vi "NI VeriStand - Get All Waveforms.vi"(8 "error in":errorcluster, 11 "Section Ref in":T1 format="%.0x") -> (0 "error out":errorcluster, 2 "Waveform Refs":T1[](array[typedef]) format="%.0x", 3 "Section Ref out":T1 format="%.0x", 4 "Found":bool)   [LabVIEW 2020, in "Custom Device Utility Library.lvlib"]
doc: "Gets an array of references for all the waveforms within the custom-device section specified by <B>Section Ref in</B>.\n\nThis VI performs a depth-first deep search."
uses:
  <vilib>/NI VeriStand/Custom Device Tools/Custom Device Utility Library/Custom Device Utility Library.lvlib
  <vilib>/NI VeriStand/Custom Device API/Custom Device Item Ref.ctl
  <vilib>/NI VeriStand/Custom Device API/Custom Device API.lvlib
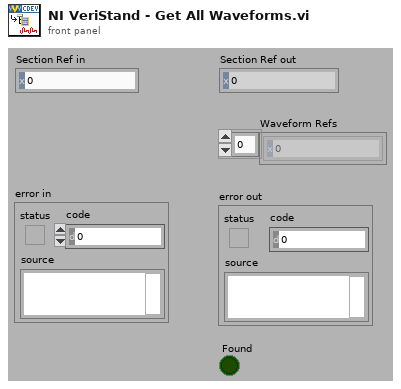
[diagram p1: front panel]
types:
  T1 = typedef "Custom Device API.lvlib/Custom Device Item Ref.ctl" = u64
  T2 = typedef "Custom Device API.lvlib/Custom Device Item Info.ctl" = cluster{"Name":string, "Is Channel":bool, "GUID":string, "Is Waveform":bool}
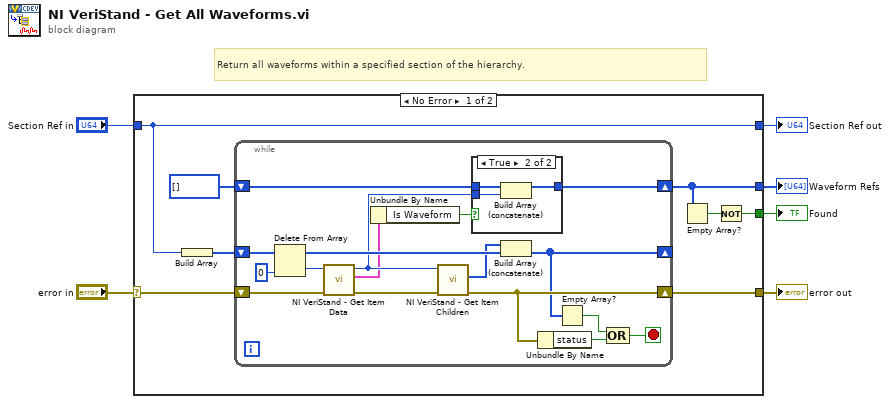
[diagram p0: block diagram]
diagram:
  # "Return all waveforms within a specified section of the hierarchy."
  n1 = case shown="No Error" "error in" {
    selector: "error in" -> [w8 w37]
    tunnel: "Section Ref in" -> [w7 w36]
    tunnel: [w13 w37] -> w5
    tunnel: [w11 _] -> w4
    tunnel: [w9 _] -> w3
    tunnel: [w7 w36] -> w1
    frame No Error {
      n2 = Build Array(w7) -> (w14:T1[])
      n3 = while {
        shift-right: [w31] -> w13
        shift-left: w8 -> [w29]
        shift-right: [w23] -> _
        shift-left: w14 -> [w28]
        shift-right: [w18] -> w11
        shift-left: T1[] [] ("appended array") -> [w19]
        stop <- w20 stop-if-true
        n4 = Delete From Array(array=w28, index=0) -> (deleted portion=w26:T1, array with subset deleted=w25:T1[])  [unwired: 1 in]
        n5 = call <vilib>:"NI VeriStand - Get Item Data.vi"("error in (no error)"=w29, "Item Ref in"=w26) -> ("error out"=w30:errorcluster, "Item Info"=w16:T2, "Item Ref out"=w17:T1)  [unwired: 7 out]
        n6 = Unbundle By Name(w16) -> ("Is Waveform"=w15:bool)
        n7 = call <vilib>:"NI VeriStand - Get Item Children.vi"("error in (no error)"=w30, "Item Ref in"=w17) -> ("error out"=w31:errorcluster, "Child Refs"=w24:T1[])  [unwired: 8 out]
        n8 = case shown="True" w15 {
          tunnel: w19 -> [w32 w35]
          tunnel: [w32 w34] -> w18
          tunnel: w17 -> [_ w33]
          frame False {
          }
          frame True {
            n9 = Build Array (concatenate)(w35, w33) -> (w34:T1[])
          }
        }
        n10 = Build Array (concatenate)(w24, w25) -> (w23:T1[])
        n11 = Unbundle By Name(w31) -> ("status"=w22:bool)
        n12 = Empty Array?(array=w23) -> (empty?=w21:bool)
        n13 = Compound Arithmetic op=OR(w21, w22) -> (w20:bool)
      }
      n14 = Empty Array?(array=w11) -> (empty?=w10:bool)
      n15 = Not(x=w10) -> (.not. x?=w9:bool)
    }
    frame Error {
    }
  }
  "Found" <- w3
  "error out" <- w5
  "Section Ref out" <- w1
  "Waveform Refs" <- w4
